vi "removeShortMeasurement.vi"(8 "error in (no error)":errorcluster, 10 "Queue in":T4, 11 "SHIFTER DATA":T1) -> (0 "error out":errorcluster)   [LabVIEW 2013, in "main.lvlib"]
uses:
  main.lvlib
  Components/Dependencies.llb/amc_Message Queue.ctl
  Components/Dependencies.llb/amc_Message.ctl
  <vilib>/FTP/util/Keyed Array.ctl
  Components/TypeDef - SHIFTER.ctl
  Components/Dependencies.llb/Exit Event Ref.ctl
  New Design/Controls/Reference Cluster.ctl
  <vilib>/Utility/sysdir.llb/System Directory Type.ctl
  Globals/DataAcqRecordPathGlobal.vi
  <userlib>/_OpenG.lib/file/file.llb/File Exists - Scalar__ogtk.vi
  Components/Dependencies.llb/TLB_Dependencies.lvlib
  <vilib>/FTP/NI_FTP.lvlib
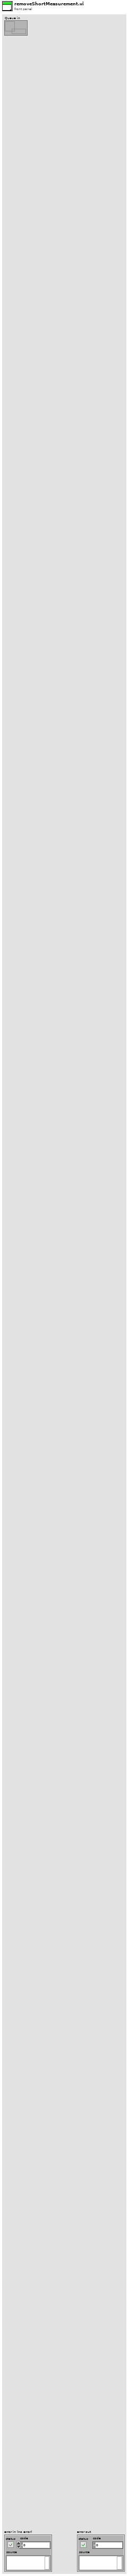
[diagram p1: front panel]
types:
  T1 = typedef "main.lvlib/TypeDef - SHIFTER.ctl" = cluster{"Exit Event":T2, "Terminate Error":errorcluster, "User Parameter Controls":refnum<vi>[], "User Parameters":cluster{"Name":string, "CPR Number":string, "Measuring Type ":string, "Measuring Technique":string, "Measuring Limb":string, "Operator":string, "Doctor":string, "Comment":string, "AdditionalInfo":string, "RightArm":string[][], "LeftArm":string[][], "PalpationRight":string, "PalpationLeft":string, "Puls":dbl, "Temp One":dbl, "Temp Two":dbl, "ActivityBox":bool}, "System Parameters":cluster{"Paper Running?":bool, "GraphSelection":bool, "Date":string, "Active Page":string}, "Data Acquisition":cluster{"Acquisition":bool, "DAQmx Task":refnum<k21>, "DAQmx Error":errorcluster, "Record number":dbl, "RecordPath":path, "AcqDataRef":refnum<vi>, "Duration":timestamp, "Queue":refnum<queue>, "Control?":bool, "RelativeRecordPath":path}, "Reference signal":cluster{"DAQmx  Task ":refnum<k21>, "Monitor":bool, "Events":dbl, "Time":timestamp, "NullEvents":dbl, "RefDataRef":refnum<vi>, "Queue":refnum<queue>}, "Data Process":cluster{"SubpanelRef":refnum<vi>, "ActiveItemTag":string, "Queue":refnum<queue>}, "System Parameter Controls":refnum<vi>[], "Database":cluster{"PatientdataRef":refnum<file>, "PatientdataPath":path, "Blue Pressure":dbl, "Red Pressure":dbl, "ActiveItemTag":string, "Height Adjustment":dbl, "BluePositionArray":dbl[][], "RedPositionArray":dbl[][], "JournalPath":path}, "MWL":cluster{"PatientID":string, "Name":string, "DICOM Info":path, "DICOM Variables":string[], "Worklist":string[][]}, "Control":cluster{"Queue":refnum<queue>, "SignalCluster":cluster{"Pump":bool, "Finger":bool, "Ankle":bool, "Fast Def":bool, "Slow Def":bool, "Init Cal":bool, "Table Pres":bool, "Table":bool}}, "PageMenu":cluster{"VI Reference":refnum<vi>, "Queue":refnum<queue>}, "Profile":cluster{"VI Reference":refnum<vi>, "Queue":refnum<queue>}, "Configuration":cluster{"VI Reference":refnum<vi>, "Queue":refnum<queue>}, "Acquisition":cluster{"VI Reference":refnum<vi>, "Queue":refnum<queue>}, "Data":cluster{"VI Reference":refnum<vi>, "Queue":refnum<queue>}, "Journal":cluster{"VI Reference":refnum<vi>, "Queue":refnum<queue>}, "cRef":T3, "Bluetooth":cluster{"Queue":refnum<queue>, "VI Reference":refnum<vi>}}
  T2 = typedef "main.lvlib/TLB_Dependencies.lvlib/Exit Event Ref.ctl" = refnum<user-event>
  T3 = typedef "main.lvlib/Reference Cluster.ctl" = cluster{"Menu":cluster{"References":cluster{"Stop Acq":refnum<vi>, "MenuExit":refnum<vi>, "MenuStartADC":refnum<vi>, "PersonalInfoString":refnum<vi>, "Profile":refnum<vi>, "Configuration":refnum<vi>, "Acquisition":refnum<vi>, "Data":refnum<vi>, "Journal":refnum<vi>}}, "Profile":cluster{"References":cluster{"Search Patient ID":refnum<vi>, "Name":refnum<vi>, "CommentStr":refnum<vi>, "Listbox Patient ID":refnum<vi>, "ListboxDoctor":refnum<vi>, "ListboxOperator":refnum<vi>, "HospitalName":refnum<vi>, "HospitalDepartment":refnum<vi>, "HospitalAddress":refnum<vi>, "EditHospInfo":refnum<vi>, "Add Patient ID Btn":refnum<vi>, "Query Worklist":refnum<vi>}}, "Configuration":cluster{"References":cluster{"ListboxMeasurementArea":refnum<vi>, "ListboxMeasurementTechnique":refnum<vi>, "ListboxMeasurementMeth":refnum<vi>, "ListboxRightSegmentNr":refnum<vi>, "ListboxLeftSegmentNr":refnum<vi>, "HeightAdjustmentInt":refnum<vi>, "PalpationRight":refnum<vi>, "PalpationLeft":refnum<vi>, "ActivityBox":refnum<vi>}, "New method":cluster{"AddNewMeasurementBtn":refnum<vi>, "Left Time Table":refnum<vi>, "Right Time Table":refnum<vi>}, "Old method":cluster{"LeftArmPressureTable":refnum<vi>, "RightArmPressureTable":refnum<vi>, "SaveArmPressureBtn":refnum<vi>, "Puls":refnum<vi>, "TempTwo":refnum<vi>, "TempOne":refnum<vi>}, "Method":string}, "Acquisition":cluster{"References":cluster{"SegmentAcqString":refnum<vi>, "RingActGraph":refnum<vi>}}, "Data":cluster{"References":cluster{"cmString":refnum<vi>, "AdjustedHeight":refnum<vi>, "Menu":refnum<vi>, "Tangent On/Off":refnum<vi>, "FilterControl":refnum<vi>}}, "Journal":cluster{"References":cluster{"ReportSelection":refnum<vi>, "Data":refnum<vi>, "GenerateReport":refnum<vi>, "Menu":refnum<vi>, "Send To PACS":refnum<vi>}}}
  T4 = typedef "main.lvlib/TLB_Dependencies.lvlib/amc_Message Queue.ctl" = refnum<queue>
  T5 = typedef "System Directory Type.ctl" = i32
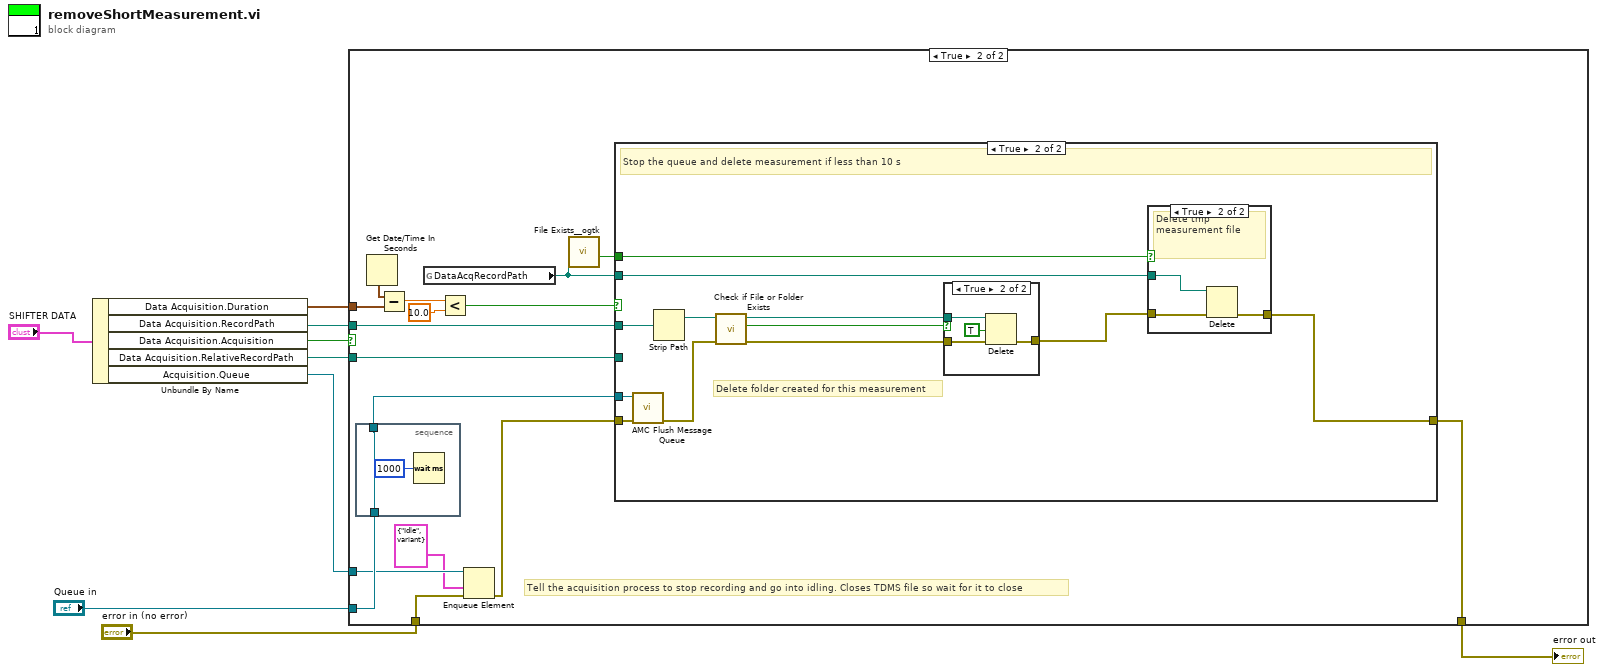
[diagram p0: block diagram]
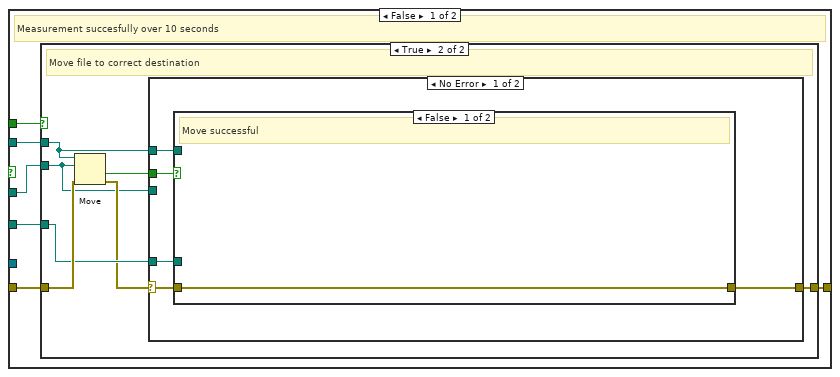
[diagram p3: hidden frame]
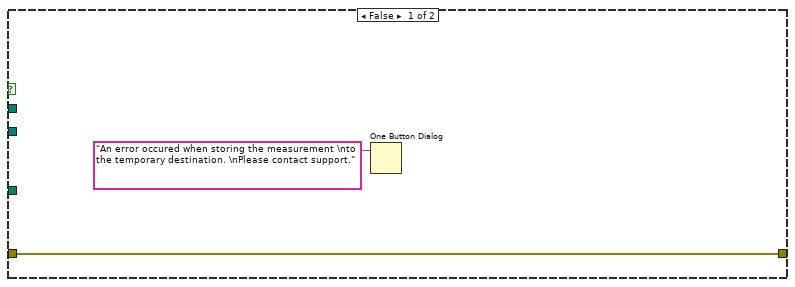
[diagram p4: hidden frame]
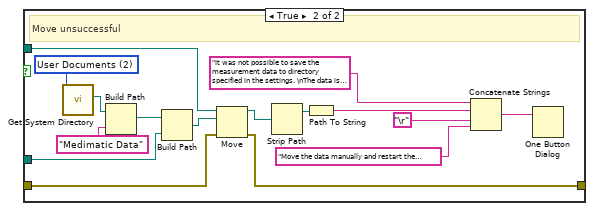
[diagram p5: hidden frame]
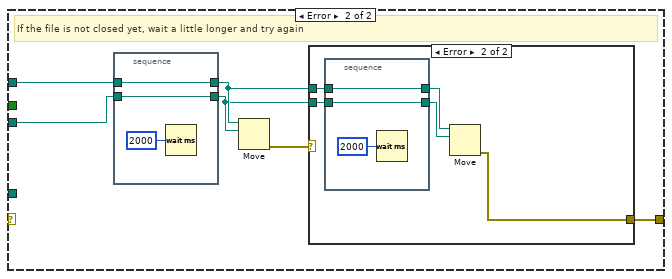
[diagram p6: hidden frame]
diagram:
  n1 = Unbundle By Name("SHIFTER DATA") -> ("Data Acquisition.Duration"=w4:timestamp, "Data Acquisition.RecordPath"=w7:path, "Data Acquisition.Acquisition"=w6:bool, "Data Acquisition.RelativeRecordPath"=w1:path, "Acquisition.Queue"=w9:refnum<queue>)
  n2 = case shown="True" w6 {
    tunnel: "error in (no error)" -> [w10 w20]
    tunnel: [w10 w15] -> w3
    tunnel: w4 -> [_ w25]
    tunnel: "Queue in" -> [_ w22]
    tunnel: w7 -> [_ w17]
    tunnel: w9 -> [_ w19]
    tunnel: w1 -> [_ w11]
    frame False {
    }
    frame True {
      # "Tell the acquisition process to stop recording and go into idling. Closes TDMS file so wait for it to close"
      n3 = stacked-sequence {
        tunnel: w22 -> [w27]
        tunnel: [w27] -> w21
        frame #0 {
          n4 = Wait (ms)(milliseconds to wait=u32 1000) -> ()  [unwired: 1 out]
        }
      }
      n5 = Get Date/Time In Seconds() -> (seconds since 1Jan1904=w26:timestamp)
      n6 = Subtract(x=w26, y=w25) -> (x-y=w24:dbl)
      n7 = global read "DataAcqRecordPathGlobal.vi" "DataAcqRecordPath"() -> (w13:path)
      n8 = Less?(x=w24, y=10.0) -> (x < y?=w14:bool)
      n9 = Enqueue Element(queue=w19, element=cluster{"Msg":string, "Data":variant} {"Msg"="Idle", "Data"=variant}, error in (no error)=w20) -> (error out=w16:errorcluster)  [unwired: 1 in, 2 out]
      n10 = call-poly <userlib>:"File Exists__ogtk.vi"("file path"=w13) -> ("exists"=w12:bool)  [unwired: 6 in, 1 out]
      n11 = case shown="True" w14 {
        tunnel: w21 -> [_ w95]
        tunnel: w17 -> [w33 w90]
        tunnel: w13 -> [w34 w93]
        tunnel: w16 -> [w32 w94]
        tunnel: [w31 w92] -> w15
        tunnel: w12 -> [w30 w91]
        tunnel: w11 -> [w29 _]
        frame False {
          # "Measurement succesfully over 10 seconds"
          n12 = case shown="True" w30 {
            tunnel: w34 -> [_ w41]
            tunnel: w33 -> [_ w37]
            tunnel: w32 -> [w35 w43]
            tunnel: [w35 w40] -> w31
            tunnel: w29 -> [_ w39]
            frame False {
              n13 = One Button Dialog(message="An error occured when storing the measurement \nto the temporary destination. \nPlease contact support.") -> ()  [unwired: 1 in, 1 out]
            }
            frame True {
              # "Move file to correct destination"
              n14 = Move(source path=w41, error in=w43, 10:w37) -> (error out=w38:errorcluster, 1:w42:bool)  [unwired: 2 in, 1 out]
              n15 = case shown="No Error" w38 {
                selector: w38 -> [w44 _]
                tunnel: w42 -> [w48 _]
                tunnel: w41 -> [w47 w71]
                tunnel: [w46 w66] -> w40
                tunnel: w39 -> [w45 _]
                tunnel: w37 -> [_ w70]
                frame No Error {
                  n16 = case shown="False" w48 {
                    tunnel: w47 -> [_ w60]
                    tunnel: w44 -> [w49 w58]
                    tunnel: [w49 w57] -> w46
                    tunnel: w45 -> [_ w61]
                    frame False {
                      # "Move successful"
                    }
                    frame True {
                      w63 = T5 2 items=["User Home"=0, "User Desktop"=1, "User Documents"=2, "User Application Data"=3, "User Preferences"=4, "User Temporary"=5, "Public Documents"=6, "Public Application Data"=7, "Public Preferences"=8, "Public Cache"=13, "System Core Libraries"=9, "System Installed Libraries"=10, "Application Files"=11, "Boot Volume Root"=12] ("system directory type")
                      # "Move unsuccessful"
                      n17 = call <vilib>:"Get System Directory.vi"("system directory type"=w63) -> ("system directory"=w65:path)  [unwired: 10 in]
                      n18 = Build Path(base path=w65, name or relative path="Medimatic Data") -> (appended path=w62:path)
                      n19 = Build Path(base path=w62, name or relative path=w61) -> (appended path=w59:path)
                      n20 = Move(source path=w60, error in=w58, 10:w59) -> (error out=w57:errorcluster, 3:w55:path)  [unwired: 2 in, 1 out]
                      n21 = Strip Path(path=w55) -> (stripped path=w54:path)  [unwired: 1 out]
                      n22 = Path To String(path=w54) -> (string=w53:string)
                      n23 = Concatenate Strings("It was not possible to save the measurement data to directory specified in the settings. \nThe data is stored in a temporary location: ", w53, "\r", "Move the data manually and restart the program when you gain access.") -> (w50:string)
                      n24 = One Button Dialog(message=w50) -> ()  [unwired: 1 in, 1 out]
                    }
                  }
                }
                frame Error {
                  # "If the file is not closed yet, wait a little longer and try again"
                  n25 = stacked-sequence {
                    tunnel: w71 -> [w82]
                    tunnel: w70 -> [w81]
                    tunnel: [w82] -> w68
                    tunnel: [w81] -> w67
                    frame #0 {
                      n26 = Wait (ms)(milliseconds to wait=u32 2000) -> ()  [unwired: 1 out]
                    }
                  }
                  n27 = Move(source path=w68, 10:w67) -> (error out=w69:errorcluster)  [unwired: 3 in, 2 out]
                  n28 = case shown="Error" w69 {
                    selector: w69 -> [w72 _]
                    tunnel: w68 -> [_ w75]
                    tunnel: w67 -> [_ w74]
                    tunnel: [w72 w73] -> w66
                    frame No Error {
                    }
                    frame Error {
                      n29 = stacked-sequence {
                        tunnel: w75 -> [w79]
                        tunnel: w74 -> [w78]
                        tunnel: [w79] -> w77
                        tunnel: [w78] -> w76
                        frame #0 {
                          n30 = Wait (ms)(milliseconds to wait=u32 2000) -> ()  [unwired: 1 out]
                        }
                      }
                      n31 = Move(source path=w77, 10:w76) -> (error out=w73:errorcluster)  [unwired: 3 in, 2 out]
                    }
                  }
                }
              }
            }
          }
        }
        frame True {
          # "Delete folder created for this measurement"
          # "Stop the queue and delete measurement if less than 10 s"
          n32 = call "AMC Flush Message Queue.vi"("error in (no error)"=w94, "Message Queue in"=w95) -> ("error out"=w88:errorcluster)  [unwired: 7 in, 1 out]
          n33 = Strip Path(path=w90) -> (stripped path=w89:path)  [unwired: 1 out]
          n34 = call <vilib>:"Check if File or Folder Exists.vi"("error in (no error)"=w88, "path"=w89) -> ("error out"=w85:errorcluster, "file or folder exists?"=w87:bool, "dup path"=w86:path)  [unwired: 7 in]
          n35 = case shown="True" w87 {
            tunnel: w86 -> [_ w100]
            tunnel: w85 -> [w96 w98]
            tunnel: [w96 w99] -> w84
            frame False {
            }
            frame True {
              # "Delete tmp measurement file"
              n36 = Delete(path (use dialog)=w100, entire hierarchy (F)=TRUE, error in=w98) -> (error out=w99:errorcluster)  [unwired: 2 in, 2 out]
            }
          }
          n37 = case shown="True" w91 {
            tunnel: w93 -> [_ w104]
            tunnel: w84 -> [w101 w103]
            tunnel: [w101 w102] -> w92
            frame False {
            }
            frame True {
              # "Delete tmp measurement file"
              n38 = Delete(path (use dialog)=w104, error in=w103) -> (error out=w102:errorcluster)  [unwired: 3 in, 2 out]
            }
          }
        }
      }
    }
  }
  "error out" <- w3
